vi "SetDAQ_AO.vi"(6 "Index":i32, 8 "error in (no error)":errorcluster, 9 "Frecuencia":dbl, 10 "Vref":dbl, 11 "Prueba33 in":refnum<class "Prueba33.lvclass">) -> (0 "error out":errorcluster, 3 "Prueba33 out":refnum<class "Prueba33.lvclass">)   [LabVIEW 2019, in "Prueba33.lvclass"]
uses:
  Prueba33.lvclass
  Prueba33.lvclass/Prueba33.ctl
  <vilib>/DAQmx/write.llb/DAQmx Write (Analog 1D Wfm NChan NSamp).vi
  <vilib>/DAQmx/miscellaneous.llb/DAQmx Fill In Error Info.vi
  <vilib>/measure/NI_MABase.lvlib
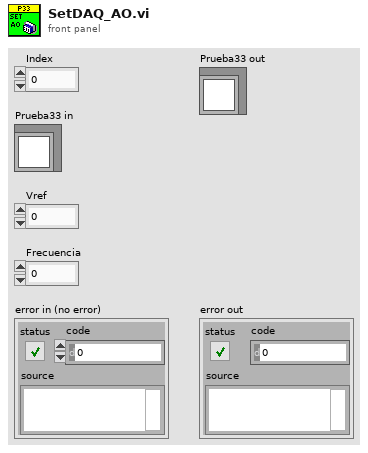
[diagram p1: front panel]
types:
  T1 = cluster{"Waveform Type":u16, "Amplitude":dbl, "Frequency":dbl}
  T2 = cluster{"Waveform Type":u16, "Amplitude":dbl, "Frequency":dbl}[]
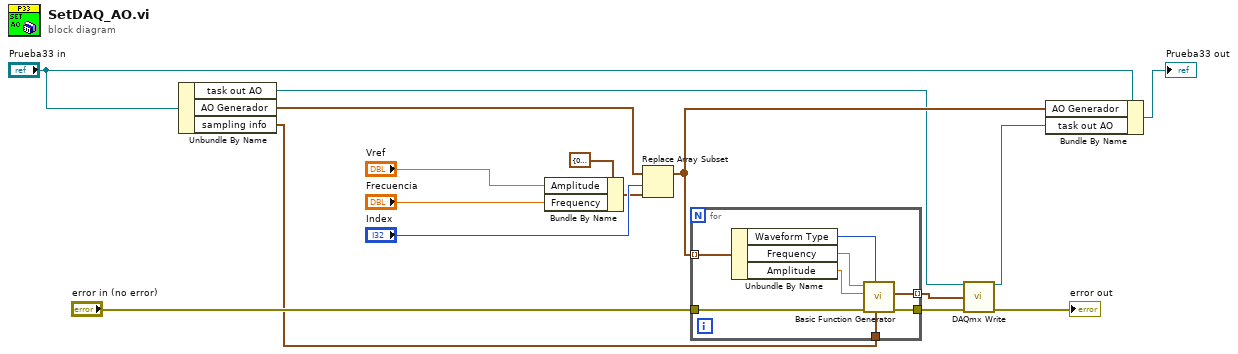
[diagram p0: block diagram]
diagram:
  n1 = Unbundle By Name("Prueba33 in") -> ("task out AO"=w1:refnum<k21>, "AO Generador"=w3:T2, "sampling info"=w2:cluster{"Fs":dbl, "#s":dbl})
  n2 = Bundle By Name(cluster=T1 {"Waveform Type"=0, "Amplitude"=1.0, "Frequency"=10.0} ("Cluster"), "Amplitude"="Vref", "Frequency"="Frecuencia") -> (w5:T1)
  n3 = Replace Array Subset(array=w3, new element=w5, index="Index") -> (w12:T2)
  n4 = for {
    tunnel: w2 -> [w24]
    tunnel: w12 -> [w23] mode=indexing
    tunnel: [w19] -> w16 mode=indexing
    tunnel: "error in (no error)" -> [w18]
    tunnel: [w17] -> w10
    n5 = Unbundle By Name(w23) -> ("Waveform Type"=w22:u16, "Frequency"=w21:dbl, "Amplitude"=w20:dbl)
    n6 = call <vilib>:"Basic Function Generator.vi"("sampling info"=w24, "signal type"=w22, "error in (no error)"=w18, "amplitude"=w20, "frequency"=w21) -> ("error out"=w17:errorcluster, "signal out"=w19:waveform(dbl))  [unwired: 4 in, 1 out]
  }
  n7 = call-poly <vilib>:"DAQmx Write.vi"("task/channels in"=w1, "data"=w16, "error in"=w10) -> ("task out"=w15:refnum<k21>, "error out"=→"error out":errorcluster)  [unwired: 10 in, 1 out]
  n8 = Bundle By Name(cluster="Prueba33 in", "AO Generador"=w12, "task out AO"=w15) -> (→"Prueba33 out":refnum<class "Prueba33.lvclass">)
